vi "Encode Signature.vi"(7 "HASH-method":T1=enum."SHA-1", 8 "error in (no error)":errorcluster, 9 "Signature Base string":string, 10 "consumer secret":string, 11 "token secret":string) -> (0 "error out":errorcluster, 2 "Encoded Signature":string)   [LabVIEW 2011, in "i3-oauth.lvlib"]
uses:
  i3-oauth.lvlib
  i3-external-encryption/labviewencryption/hash-types.ctl
  i3-external-encryption/i3-external-encryption.lvlib
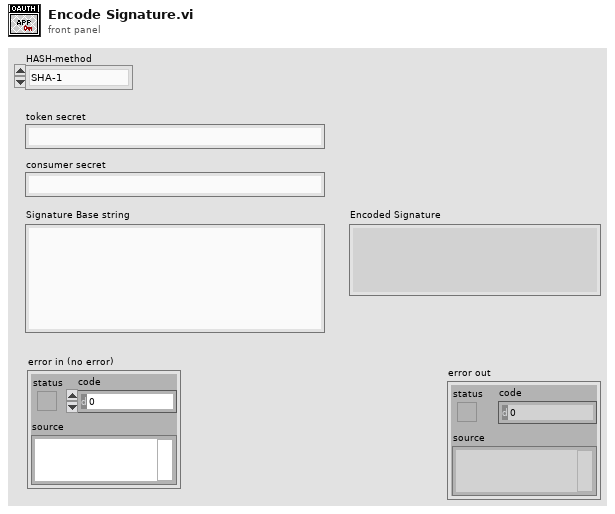
[diagram p1: front panel]
types:
  T1 = typedef "i3-external-encryption.lvlib/hash-types.ctl" = enum16{"MD5", "SHA-1", "SHA-224", "SHA-256", "SHA-384", "SHA-512"}
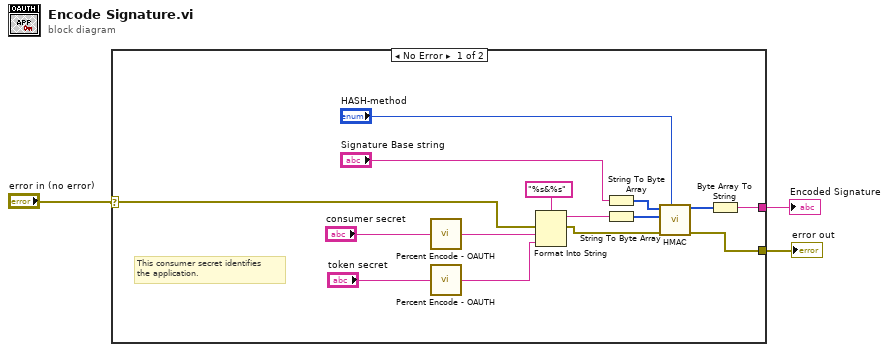
[diagram p0: block diagram]
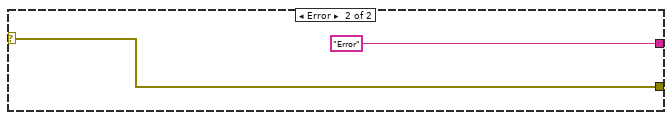
[diagram p2: hidden frame]
diagram:
  n1 = case shown="No Error" "error in (no error)" {
    selector: "error in (no error)" -> [w5 w20]
    tunnel: [w8 "Error"] -> w3
    tunnel: [w6 w20] -> w2
    frame No Error {
      # "This consumer secret identifies\nthe application."
      n2 = call "Percent Encode - OAUTH.vi"("unescaped string in"="consumer secret") -> ("escaped string out"=w17:string)
      n3 = call "Percent Encode - OAUTH.vi"("unescaped string in"="token secret") -> ("escaped string out"=w16:string)
      n4 = Format Into String(format string="%s&%s", error in=w5, w17, w16) -> (resulting string=w10:string, error out=w7:errorcluster)  [unwired: 1 in]
      n5 = String To Byte Array(string="Signature Base string") -> (unsigned byte array=w14:u8[])
      n6 = String To Byte Array(string=w10) -> (unsigned byte array=w13:u8[])
      n7 = call "HMAC.vi"("HASH-method"="HASH-method", "error in (no error)"=w7, "Key"=w13, "Message"=w14) -> ("error out"=w6:errorcluster, "HMAC digest"=w12:u8[])  [unwired: 5 in, 1 out]
      n8 = Byte Array To String(unsigned byte array=w12) -> (string=w8:string)
    }
    frame Error {
    }
  }
  "error out" <- w2
  "Encoded Signature" <- w3
